vi "USB_TC-08 - Data table 2inputs.vi"() -> ()   [LabVIEW 2018]
uses:
  Instance           1 17Saved   USB_TC-08 .vi
  Program Files (x86)/Pico Technology/SDK/lib/usbtc08.dll
panel:
  in  "Units 3":enum16{"--"}(ring)
  in  "Units 2":enum16{"C°", "F°", "K°", "R°"}(ring)
  out "Temperature 2":dynamicdata(graph)
  in  "Type # 2.8":i16(ring)=107 items=["B"=98, "E"=101, "J"=106, "K"=107, "N"=110, "R"=114, "S"=115, "T"=116, "Voltage"=120]
  in  "Type # 2.7":i16(ring)=107 items=["B"=98, "E"=101, "J"=106, "K"=107, "N"=110, "R"=114, "S"=115, "T"=116, "Voltage"=120]
  in  "Type # 2.6":i16(ring)=107 items=["B"=98, "E"=101, "J"=106, "K"=107, "N"=110, "R"=114, "S"=115, "T"=116, "Voltage"=120]
  in  "Type # 2.5":i16(ring)=107 items=["B"=98, "E"=101, "J"=106, "K"=107, "N"=110, "R"=114, "S"=115, "T"=116, "Voltage"=120]
  in  "Type # 2.4":i16(ring)=107 items=["B"=98, "E"=101, "J"=106, "K"=107, "N"=110, "R"=114, "S"=115, "T"=116, "Voltage"=120]
  in  "Type # 2.3":i16(ring)=107 items=["B"=98, "E"=101, "J"=106, "K"=107, "N"=110, "R"=114, "S"=115, "T"=116, "Voltage"=120]
  in  "Type # 2.2":i16(ring)=107 items=["B"=98, "E"=101, "J"=106, "K"=107, "N"=110, "R"=114, "S"=115, "T"=116, "Voltage"=120]
  in  "Type # 2.1":i16(ring)=107 items=["B"=98, "E"=101, "J"=106, "K"=107, "N"=110, "R"=114, "S"=115, "T"=116, "Voltage"=120]
  in  "Ch # 2.8":bool
  in  "Ch # 2.7":bool
  in  "Ch # 2.6":bool
  in  "Ch # 2.5":bool
  in  "Ch # 2.4":bool
  in  "Ch # 2.3 2":bool
  in  "Ch# 2.2 2":bool=TRUE
  in  "Ch# 2.1":bool=TRUE
  in  "Mains Frequency 2":i16(ring) items=["50 Hz", "60 Hz"]
  out "Handle 2":i16
  in  "?":bool
  in  "Save File Path":path
  in  "Comment":string="WRITE THE COMMENT BEFORE RUNNING VI"
  in  "Save to File":bool
  out "Output Data":string[][](table)
  in  "Mains Frequency":i16(ring) items=["50 Hz", "60 Hz"]
  out "Temperature":dynamicdata(graph)
  in  "?":bool
  in  "Ch # 1.8":bool
  in  "Type # 1.8":i16(ring)=107 items=["B"=98, "E"=101, "J"=106, "K"=107, "N"=110, "R"=114, "S"=115, "T"=116, "Voltage"=120]
  in  "Ch # 1.7":bool
  in  "Type # 1.7":i16(ring)=107 items=["B"=98, "E"=101, "J"=106, "K"=107, "N"=110, "R"=114, "S"=115, "T"=116, "Voltage"=120]
  in  "Ch # 1.6":bool
  in  "Type # 1.6":i16(ring)=107 items=["B"=98, "E"=101, "J"=106, "K"=107, "N"=110, "R"=114, "S"=115, "T"=116, "Voltage"=120]
  in  "Ch # 1.5":bool
  in  "Type # 1.5":i16(ring)=107 items=["B"=98, "E"=101, "J"=106, "K"=107, "N"=110, "R"=114, "S"=115, "T"=116, "Voltage"=120]
  in  "Ch # 1.4":bool
  in  "Type # 1.4":i16(ring)=107 items=["B"=98, "E"=101, "J"=106, "K"=107, "N"=110, "R"=114, "S"=115, "T"=116, "Voltage"=120]
  in  "Ch # 1.3":bool
  in  "Type # 1.3":i16(ring)=107 items=["B"=98, "E"=101, "J"=106, "K"=107, "N"=110, "R"=114, "S"=115, "T"=116, "Voltage"=120]
  in  "Ch# 1.2":bool=TRUE
  in  "Type # 1.2":i16(ring)=107 items=["B"=98, "E"=101, "J"=106, "K"=107, "N"=110, "R"=114, "S"=115, "T"=116, "Voltage"=120]
  in  "Ch# 1.1":bool=TRUE
  in  "Type # 1.1":i16(ring)=107 items=["B"=98, "E"=101, "J"=106, "K"=107, "N"=110, "R"=114, "S"=115, "T"=116, "Voltage"=120]
  in  "Units":enum16{"C°", "F°", "K°", "R°"}(ring)
  in  "stop":bool
  out "Handle":i16
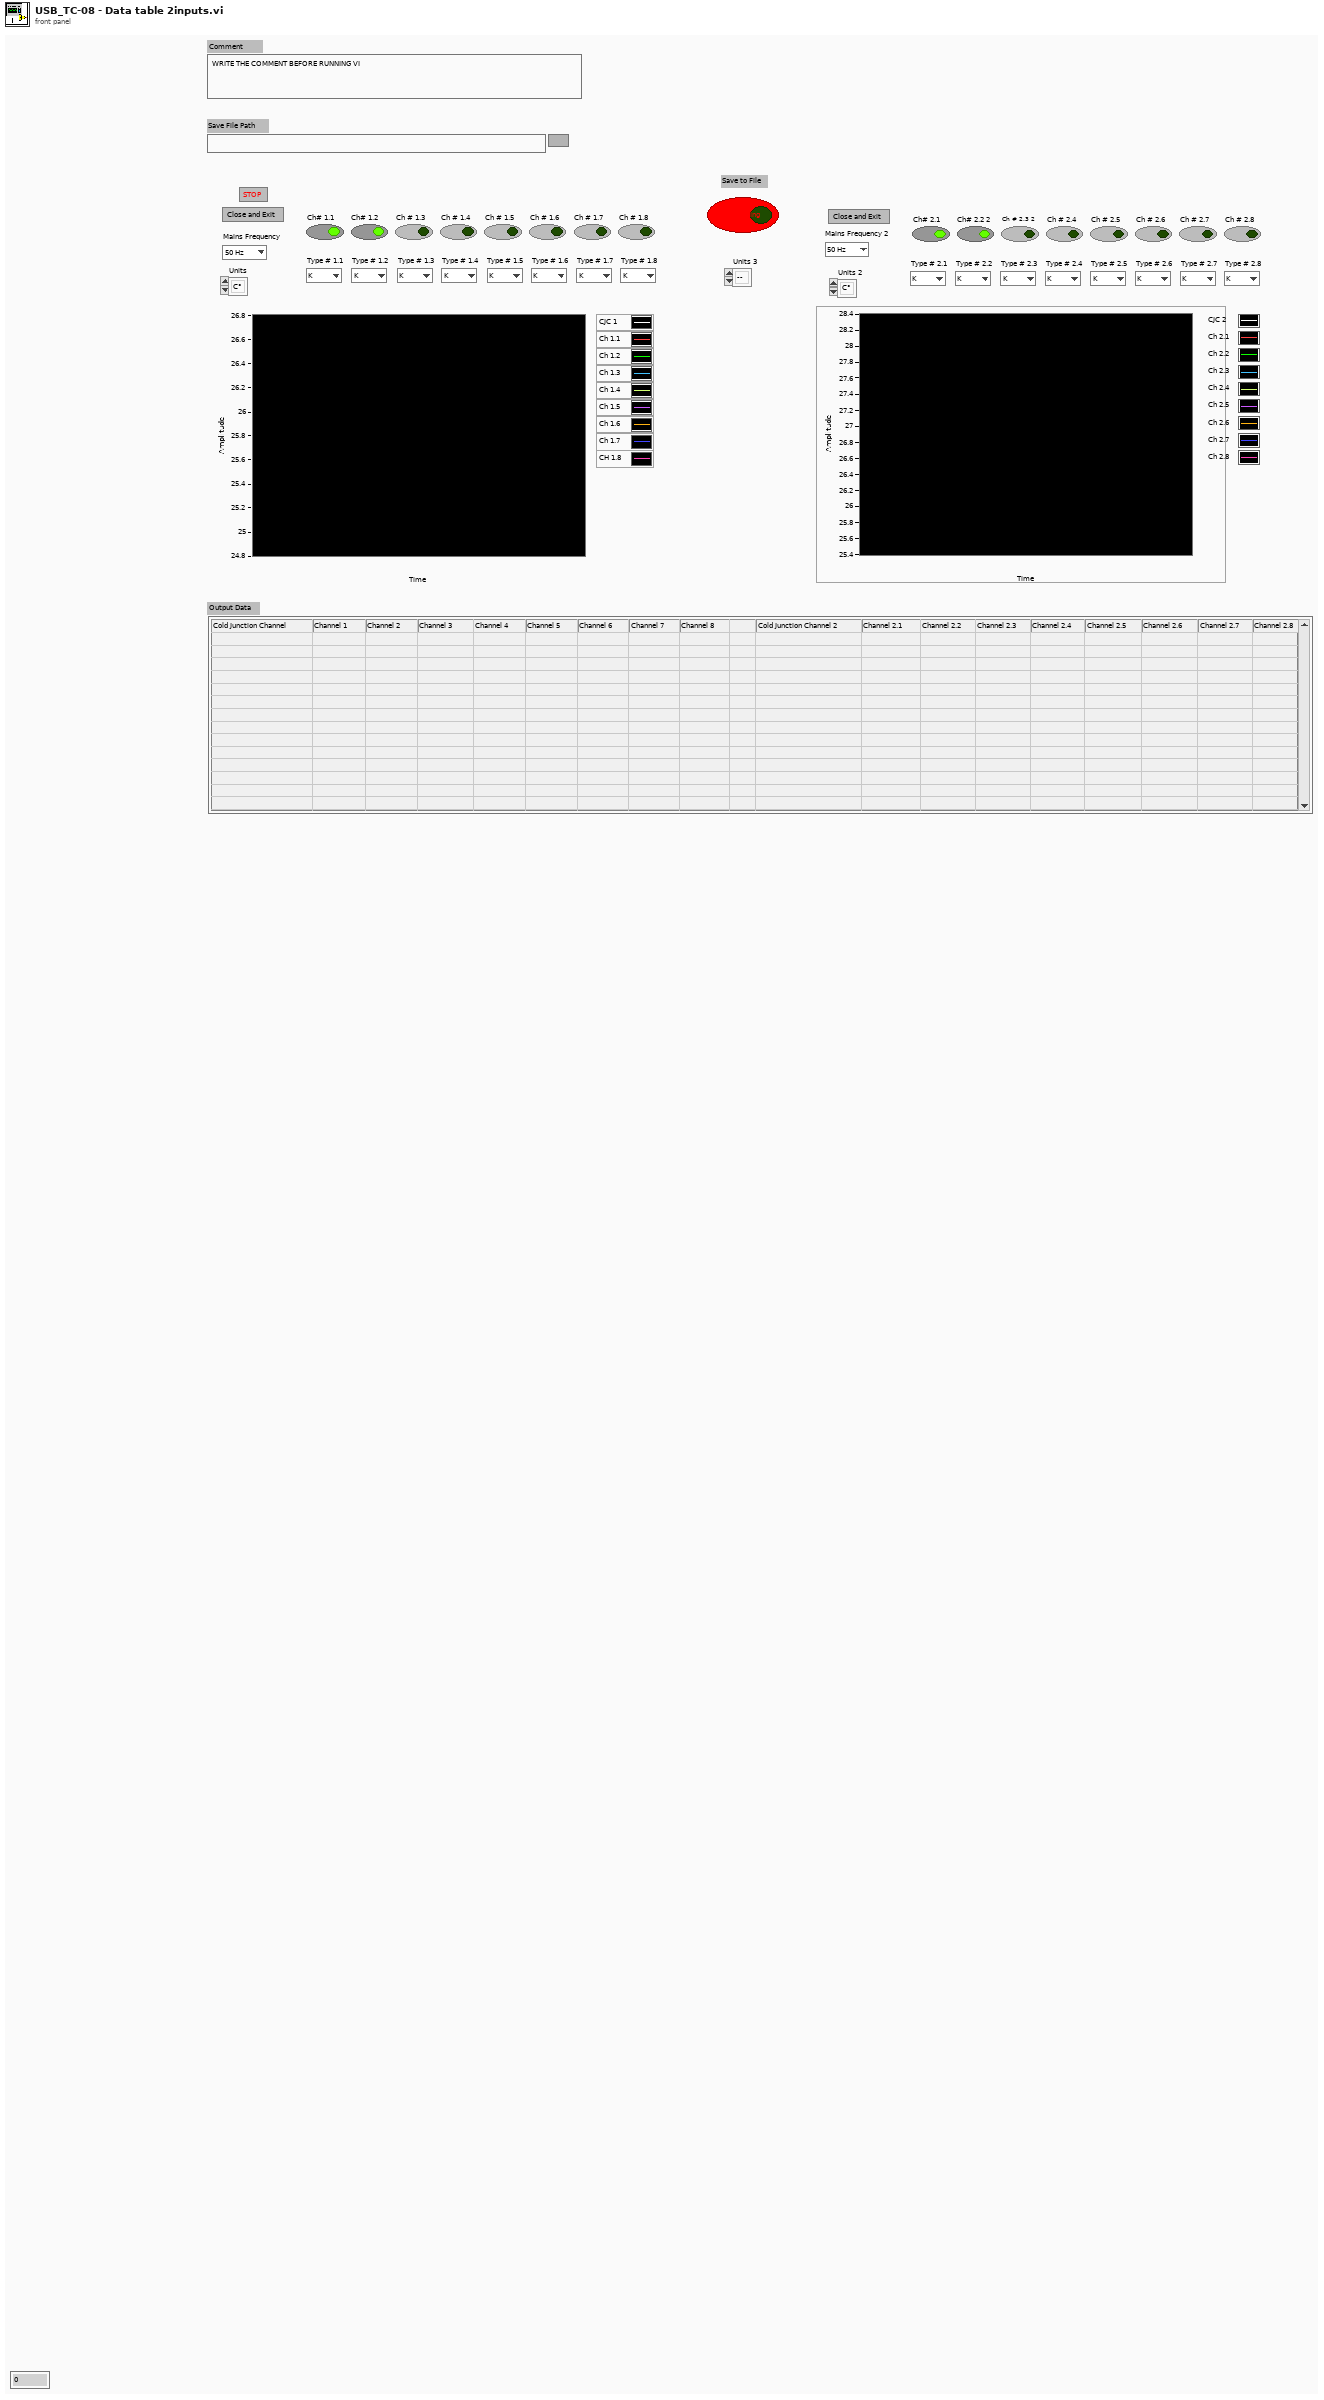
[diagram p1: front panel]
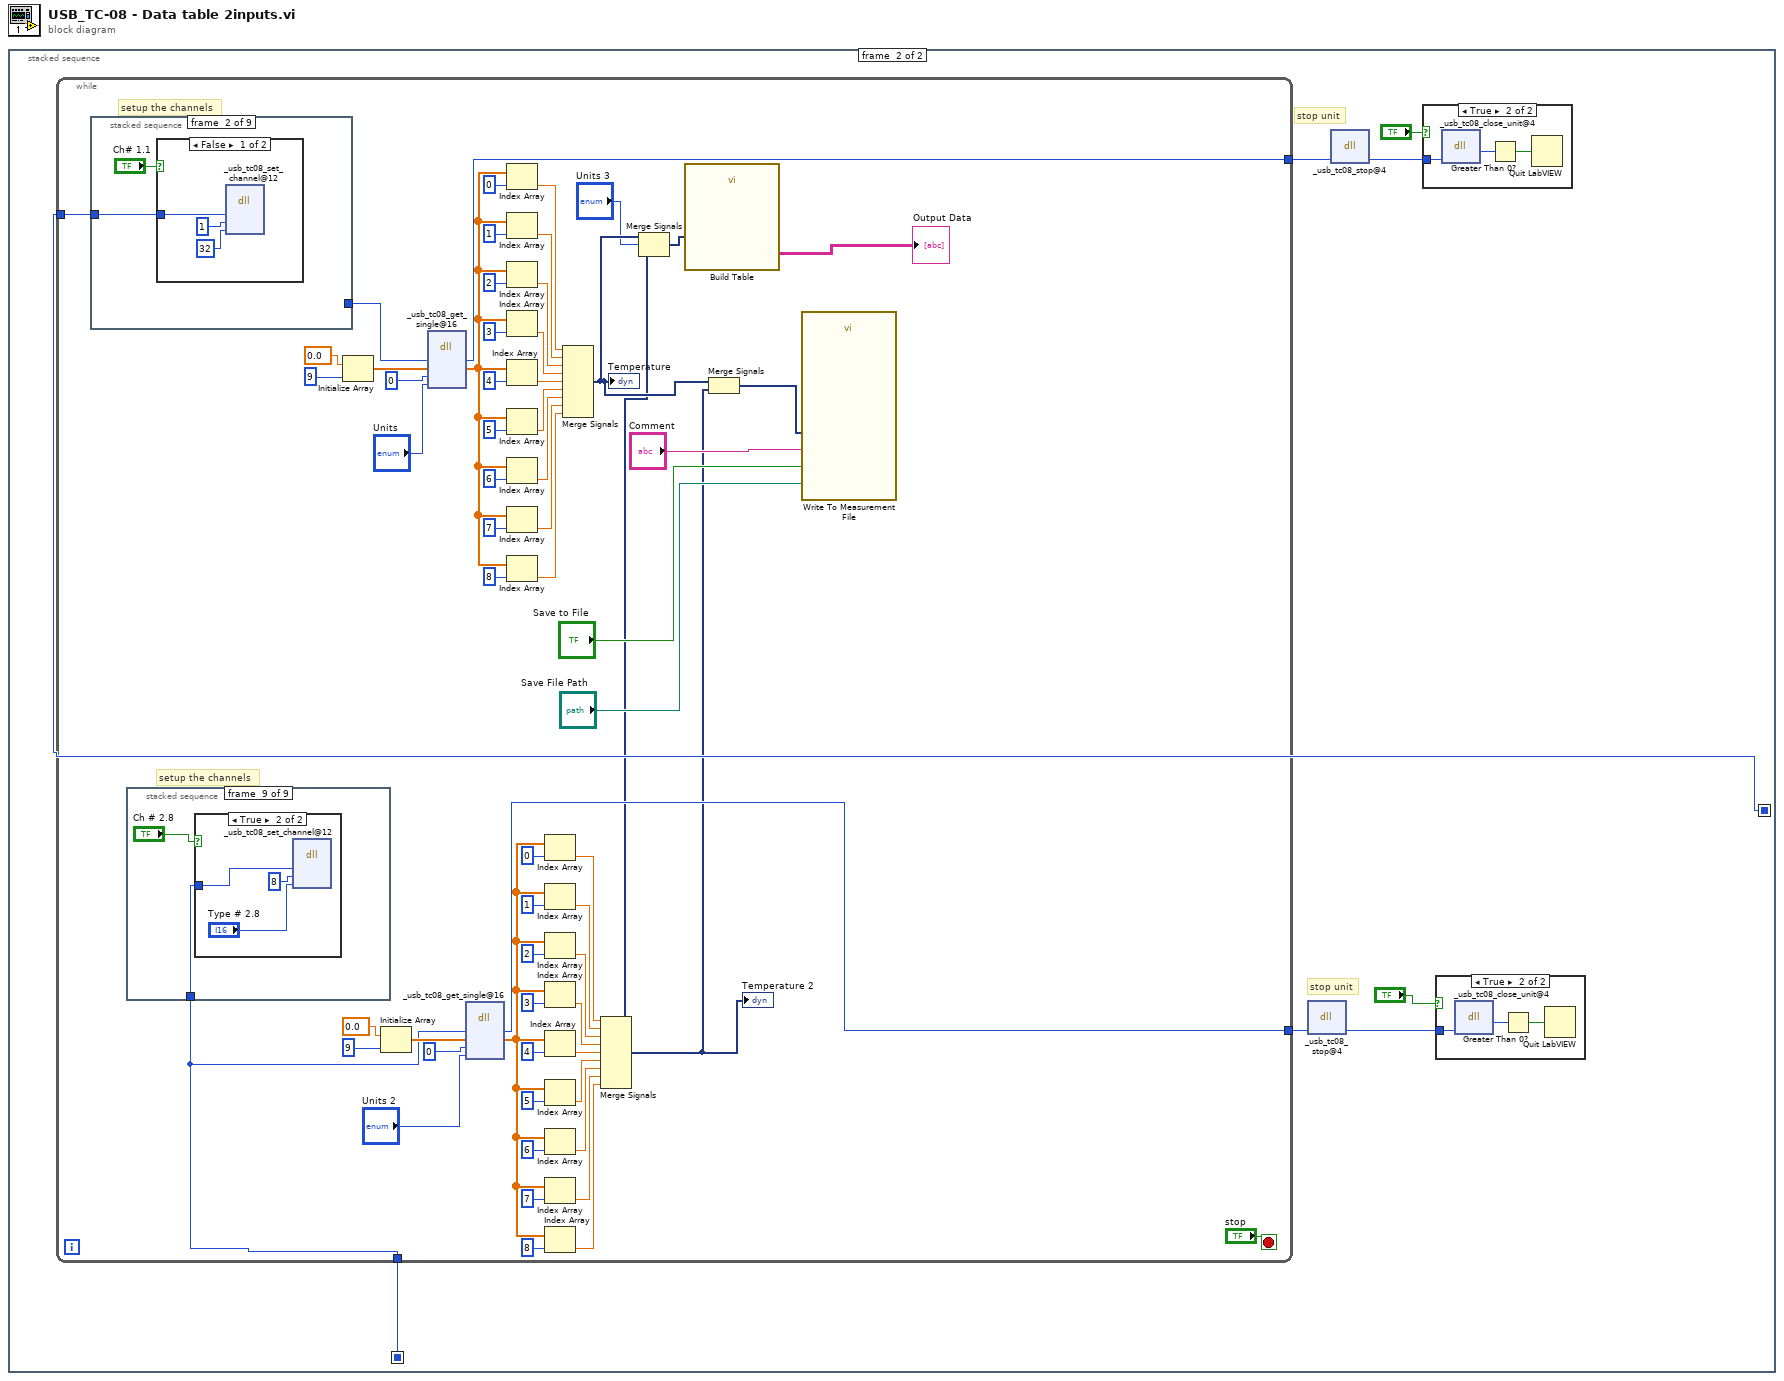
[diagram p0: block diagram]
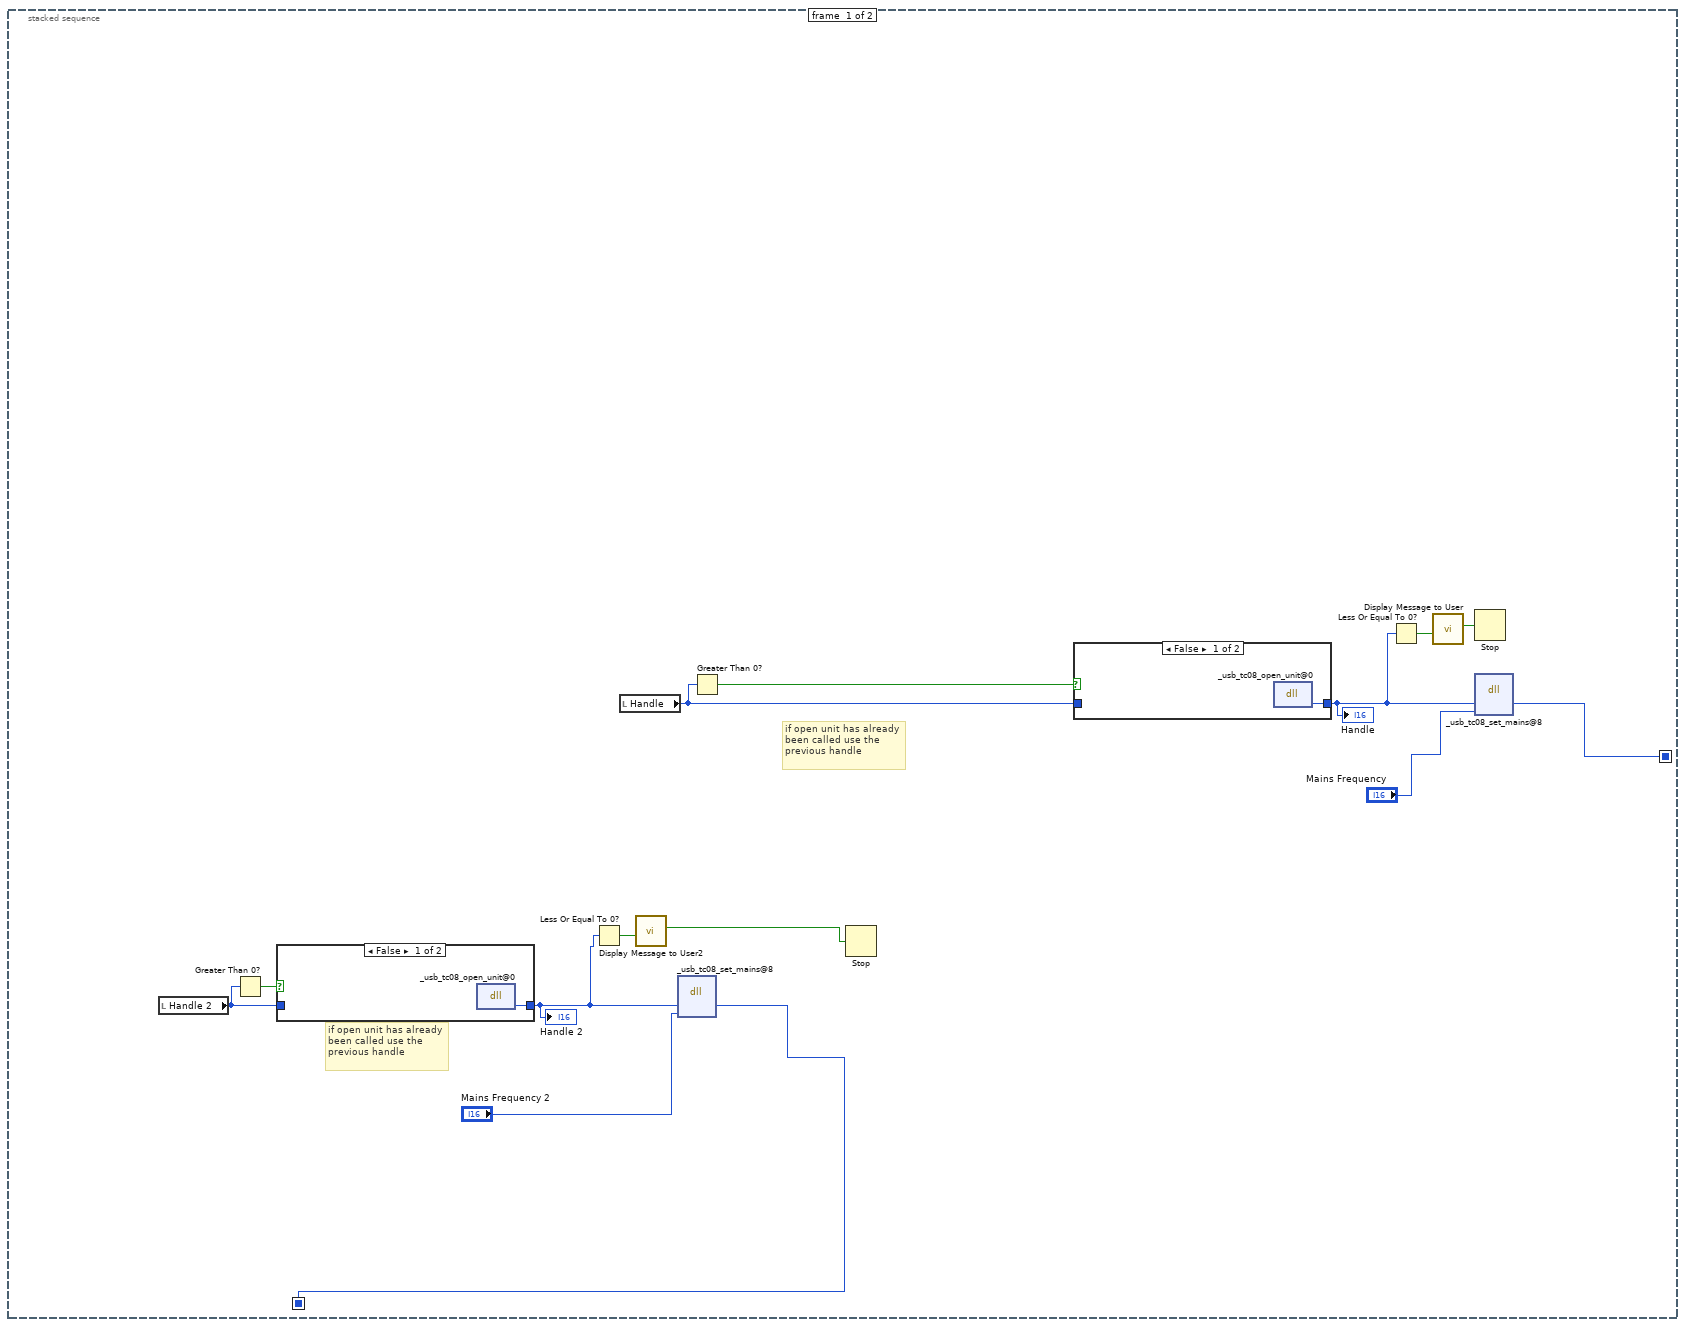
[diagram p2: hidden frame]
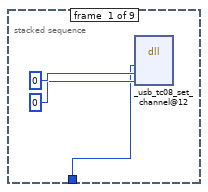
[diagram p6: hidden frame]
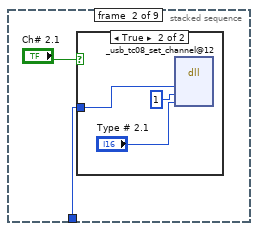
[diagram p7: hidden frame]
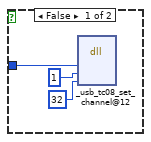
[diagram p8: hidden frame]
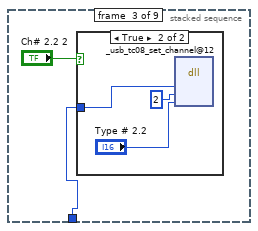
[diagram p9: hidden frame]
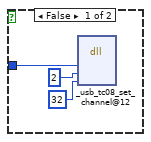
[diagram p10: hidden frame]
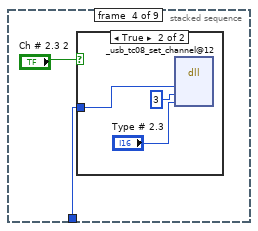
[diagram p11: hidden frame]
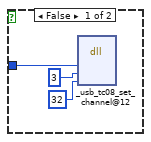
[diagram p12: hidden frame]
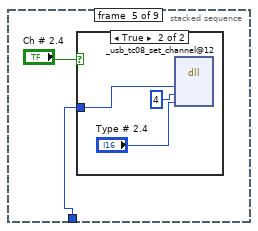
[diagram p13: hidden frame]
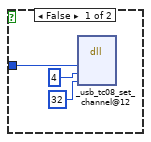
[diagram p14: hidden frame]
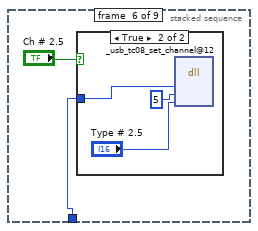
[diagram p15: hidden frame]
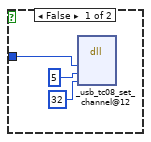
[diagram p16: hidden frame]
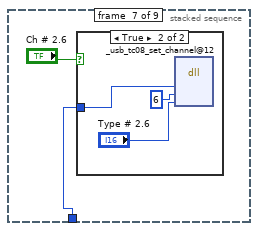
[diagram p17: hidden frame]
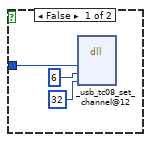
[diagram p18: hidden frame]
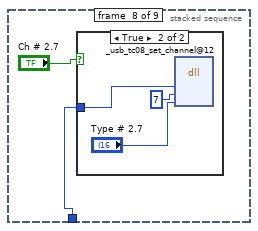
[diagram p19: hidden frame]
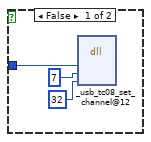
[diagram p20: hidden frame]
diagram:
  n1 = stacked-sequence {
    seq-local: [w12 _] -> [_ w23]
    seq-local: [w1 _] -> [_ w19]
    frame #0 {
      # "if open unit has already been called use the previous handle"
      # "if open unit has already been called use the previous handle"
      n2 = local read "Handle 2"() -> (w6:i16)
      n3 = Greater Than 0?(x=w6) -> (x > 0?=w5:bool)
      n4 = case shown="False" w5 {
        tunnel: [w15 w16] -> w2
        tunnel: w6 -> [_ w16]
        frame False {
          n5 = dll-call lib="//Program Files (x86)/Pico Technology/SDK/lib/usbtc08.dll" fn="_usb_tc08_open_unit@0" label="OpenUnit"() -> ("Handle"=w15:i16)  [unwired: 3 in, 2 out]
        }
        frame True {
        }
      }
      "Handle 2" <- w2
      n6 = Less Or Equal To 0?(x=w2) -> (x <= 0?=w4:bool)
      n7 = local read "Handle"() -> (w13:i16)
      n8 = call "Display Message to User2"("Enable"=w4) -> ("OK"=w3:bool)  [unwired: 9 in, 1 out]
      n9 = dll-call lib="//Program Files (x86)/Pico Technology/SDK/lib/usbtc08.dll" fn="_usb_tc08_set_mains@8" label="Set Mains"("Handle"=w2, "sixtyHertz"="Mains Frequency 2") -> ("Handle"=w1:i16)  [unwired: 5 in, 2 out]
      n10 = Greater Than 0?(x=w13) -> (x > 0?=w14:bool)
      n11 = Stop(stop? (T)=w3) -> ()
      n12 = case shown="False" w14 {
        tunnel: [w17 w18] -> w11
        tunnel: w13 -> [_ w18]
        frame False {
          n13 = dll-call lib="//Program Files (x86)/Pico Technology/SDK/lib/usbtc08.dll" fn="_usb_tc08_open_unit@0" label="OpenUnit"() -> ("Handle"=w17:i16)  [unwired: 3 in, 2 out]
        }
        frame True {
        }
      }
      "Handle" <- w11
      n14 = Less Or Equal To 0?(x=w11) -> (x <= 0?=w10:bool)
      n15 = call "Display Message to User"("Enable"=w10) -> ("OK"=w9:bool)  [unwired: 9 in, 1 out]
      n16 = Stop(stop? (T)=w9) -> ()
      n17 = dll-call lib="//Program Files (x86)/Pico Technology/SDK/lib/usbtc08.dll" fn="_usb_tc08_set_mains@8" label="Set Mains"("Handle"=w11, "sixtyHertz"="Mains Frequency") -> ("Handle"=w12:i16)  [unwired: 5 in, 2 out]
    }
    frame #1 {
      # "stop unit"
      # "stop unit"
      n18 = while {
        tunnel: w23 -> [w92]
        tunnel: [w66] -> w24
        tunnel: [w36] -> w20
        tunnel: w19 -> [w35]
        stop <- "stop" stop-if-true
        # "setup the channels"
        # "setup the channels"
        n19 = stacked-sequence {
          tunnel: w92 -> [w162 w164 w172 w180 w188 w196 w204 w212 w219]
          tunnel: [_ _ _ _ _ _ _ _ w219] -> w88
          frame #0 {
            n20 = dll-call lib="//Program Files (x86)/Pico Technology/SDK/lib/usbtc08.dll" fn="_usb_tc08_set_channel@12"("handle"=w162, "channel"=i16 0, "tc_type"=i8 0) -> ()  [unwired: 7 in, 2 out]
          }
          frame #1 {
            n21 = case shown="False" "Ch# 1.1" {
              tunnel: w164 -> [w166 w169]
              frame False {
                n22 = dll-call lib="//Program Files (x86)/Pico Technology/SDK/lib/usbtc08.dll" fn="_usb_tc08_set_channel@12"("handle"=w166, "channel"=i16 1, "tc_type"=32) -> ()  [unwired: 7 in, 2 out]
              }
              frame True {
                n23 = dll-call lib="//Program Files (x86)/Pico Technology/SDK/lib/usbtc08.dll" fn="_usb_tc08_set_channel@12"("handle"=w169, "channel"=i16 1, "tc_type"="Type # 1.1") -> ()  [unwired: 7 in, 2 out]
              }
            }
          }
          frame #2 {
            n24 = case shown="False" "Ch# 1.2" {
              tunnel: w172 -> [w173 w177]
              frame False {
                n25 = dll-call lib="//Program Files (x86)/Pico Technology/SDK/lib/usbtc08.dll" fn="_usb_tc08_set_channel@12"("handle"=w173, "channel"=i16 2, "tc_type"=32) -> ()  [unwired: 7 in, 2 out]
              }
              frame True {
                n26 = dll-call lib="//Program Files (x86)/Pico Technology/SDK/lib/usbtc08.dll" fn="_usb_tc08_set_channel@12"("handle"=w177, "channel"=i16 2, "tc_type"="Type # 1.2") -> ()  [unwired: 7 in, 2 out]
              }
            }
          }
          frame #3 {
            n27 = case shown="True" "Ch # 1.3" {
              tunnel: w180 -> [w181 w185]
              frame False {
                n28 = dll-call lib="//Program Files (x86)/Pico Technology/SDK/lib/usbtc08.dll" fn="_usb_tc08_set_channel@12"("handle"=w181, "channel"=i16 3, "tc_type"=32) -> ()  [unwired: 7 in, 2 out]
              }
              frame True {
                n29 = dll-call lib="//Program Files (x86)/Pico Technology/SDK/lib/usbtc08.dll" fn="_usb_tc08_set_channel@12"("handle"=w185, "channel"=i16 3, "tc_type"="Type # 1.3") -> ()  [unwired: 7 in, 2 out]
              }
            }
          }
          frame #4 {
            n30 = case shown="False" "Ch # 1.4" {
              tunnel: w188 -> [w189 w193]
              frame False {
                n31 = dll-call lib="//Program Files (x86)/Pico Technology/SDK/lib/usbtc08.dll" fn="_usb_tc08_set_channel@12"("handle"=w189, "channel"=i16 4, "tc_type"=32) -> ()  [unwired: 7 in, 2 out]
              }
              frame True {
                n32 = dll-call lib="//Program Files (x86)/Pico Technology/SDK/lib/usbtc08.dll" fn="_usb_tc08_set_channel@12"("handle"=w193, "channel"=i16 4, "tc_type"="Type # 1.4") -> ()  [unwired: 7 in, 2 out]
              }
            }
          }
          frame #5 {
            n33 = case shown="False" "Ch # 1.5" {
              tunnel: w196 -> [w197 w201]
              frame False {
                n34 = dll-call lib="//Program Files (x86)/Pico Technology/SDK/lib/usbtc08.dll" fn="_usb_tc08_set_channel@12"("handle"=w197, "channel"=i16 5, "tc_type"=32) -> ()  [unwired: 7 in, 2 out]
              }
              frame True {
                n35 = dll-call lib="//Program Files (x86)/Pico Technology/SDK/lib/usbtc08.dll" fn="_usb_tc08_set_channel@12"("handle"=w201, "channel"=i16 5, "tc_type"="Type # 1.5") -> ()  [unwired: 7 in, 2 out]
              }
            }
          }
          frame #6 {
            n36 = case shown="True" "Ch # 1.6" {
              tunnel: w204 -> [w205 w209]
              frame False {
                n37 = dll-call lib="//Program Files (x86)/Pico Technology/SDK/lib/usbtc08.dll" fn="_usb_tc08_set_channel@12"("handle"=w205, "channel"=i16 6, "tc_type"=32) -> ()  [unwired: 7 in, 2 out]
              }
              frame True {
                n38 = dll-call lib="//Program Files (x86)/Pico Technology/SDK/lib/usbtc08.dll" fn="_usb_tc08_set_channel@12"("handle"=w209, "channel"=i16 6, "tc_type"="Type # 1.6") -> ()  [unwired: 7 in, 2 out]
              }
            }
          }
          frame #7 {
            n39 = case shown="False" "Ch # 1.7" {
              tunnel: w212 -> [w213 w217]
              frame False {
                n40 = dll-call lib="//Program Files (x86)/Pico Technology/SDK/lib/usbtc08.dll" fn="_usb_tc08_set_channel@12"("handle"=w213, "channel"=i16 7, "tc_type"=32) -> ()  [unwired: 7 in, 2 out]
              }
              frame True {
                n41 = dll-call lib="//Program Files (x86)/Pico Technology/SDK/lib/usbtc08.dll" fn="_usb_tc08_set_channel@12"("handle"=w217, "channel"=i16 7, "tc_type"="Type # 1.7") -> ()  [unwired: 7 in, 2 out]
              }
            }
          }
          frame #8 {
            n42 = case shown="True" "Ch # 1.8" {
              tunnel: w219 -> [w221 w225]
              frame False {
                n43 = dll-call lib="//Program Files (x86)/Pico Technology/SDK/lib/usbtc08.dll" fn="_usb_tc08_set_channel@12"("handle"=w221, "channel"=i16 8, "tc_type"=32) -> ()  [unwired: 7 in, 2 out]
              }
              frame True {
                n44 = dll-call lib="//Program Files (x86)/Pico Technology/SDK/lib/usbtc08.dll" fn="_usb_tc08_set_channel@12"("handle"=w225, "channel"=i16 8, "tc_type"="Type # 1.8") -> ()  [unwired: 7 in, 2 out]
              }
            }
          }
        }
        n45 = stacked-sequence {
          tunnel: w35 -> [w93 w97 w105 w113 w121 w129 w137 w145 w153]
          frame #0 {
            n46 = dll-call lib="//Program Files (x86)/Pico Technology/SDK/lib/usbtc08.dll" fn="_usb_tc08_set_channel@12"("handle"=w93, "channel"=i16 0, "tc_type"=i8 0) -> ()  [unwired: 7 in, 2 out]
          }
          frame #1 {
            n47 = case shown="True" "Ch# 2.1" {
              tunnel: w97 -> [w99 w102]
              frame False {
                n48 = dll-call lib="//Program Files (x86)/Pico Technology/SDK/lib/usbtc08.dll" fn="_usb_tc08_set_channel@12"("handle"=w99, "channel"=i16 1, "tc_type"=32) -> ()  [unwired: 7 in, 2 out]
              }
              frame True {
                n49 = dll-call lib="//Program Files (x86)/Pico Technology/SDK/lib/usbtc08.dll" fn="_usb_tc08_set_channel@12"("handle"=w102, "channel"=i16 1, "tc_type"="Type # 2.1") -> ()  [unwired: 7 in, 2 out]
              }
            }
          }
          frame #2 {
            n50 = case shown="True" "Ch# 2.2 2" {
              tunnel: w105 -> [w106 w110]
              frame False {
                n51 = dll-call lib="//Program Files (x86)/Pico Technology/SDK/lib/usbtc08.dll" fn="_usb_tc08_set_channel@12"("handle"=w106, "channel"=i16 2, "tc_type"=32) -> ()  [unwired: 7 in, 2 out]
              }
              frame True {
                n52 = dll-call lib="//Program Files (x86)/Pico Technology/SDK/lib/usbtc08.dll" fn="_usb_tc08_set_channel@12"("handle"=w110, "channel"=i16 2, "tc_type"="Type # 2.2") -> ()  [unwired: 7 in, 2 out]
              }
            }
          }
          frame #3 {
            n53 = case shown="True" "Ch # 2.3 2" {
              tunnel: w113 -> [w114 w118]
              frame False {
                n54 = dll-call lib="//Program Files (x86)/Pico Technology/SDK/lib/usbtc08.dll" fn="_usb_tc08_set_channel@12"("handle"=w114, "channel"=i16 3, "tc_type"=32) -> ()  [unwired: 7 in, 2 out]
              }
              frame True {
                n55 = dll-call lib="//Program Files (x86)/Pico Technology/SDK/lib/usbtc08.dll" fn="_usb_tc08_set_channel@12"("handle"=w118, "channel"=i16 3, "tc_type"="Type # 2.3") -> ()  [unwired: 7 in, 2 out]
              }
            }
          }
          frame #4 {
            n56 = case shown="True" "Ch # 2.4" {
              tunnel: w121 -> [w122 w126]
              frame False {
                n57 = dll-call lib="//Program Files (x86)/Pico Technology/SDK/lib/usbtc08.dll" fn="_usb_tc08_set_channel@12"("handle"=w122, "channel"=i16 4, "tc_type"=32) -> ()  [unwired: 7 in, 2 out]
              }
              frame True {
                n58 = dll-call lib="//Program Files (x86)/Pico Technology/SDK/lib/usbtc08.dll" fn="_usb_tc08_set_channel@12"("handle"=w126, "channel"=i16 4, "tc_type"="Type # 2.4") -> ()  [unwired: 7 in, 2 out]
              }
            }
          }
          frame #5 {
            n59 = case shown="True" "Ch # 2.5" {
              tunnel: w129 -> [w130 w134]
              frame False {
                n60 = dll-call lib="//Program Files (x86)/Pico Technology/SDK/lib/usbtc08.dll" fn="_usb_tc08_set_channel@12"("handle"=w130, "channel"=i16 5, "tc_type"=32) -> ()  [unwired: 7 in, 2 out]
              }
              frame True {
                n61 = dll-call lib="//Program Files (x86)/Pico Technology/SDK/lib/usbtc08.dll" fn="_usb_tc08_set_channel@12"("handle"=w134, "channel"=i16 5, "tc_type"="Type # 2.5") -> ()  [unwired: 7 in, 2 out]
              }
            }
          }
          frame #6 {
            n62 = case shown="True" "Ch # 2.6" {
              tunnel: w137 -> [w138 w142]
              frame False {
                n63 = dll-call lib="//Program Files (x86)/Pico Technology/SDK/lib/usbtc08.dll" fn="_usb_tc08_set_channel@12"("handle"=w138, "channel"=i16 6, "tc_type"=32) -> ()  [unwired: 7 in, 2 out]
              }
              frame True {
                n64 = dll-call lib="//Program Files (x86)/Pico Technology/SDK/lib/usbtc08.dll" fn="_usb_tc08_set_channel@12"("handle"=w142, "channel"=i16 6, "tc_type"="Type # 2.6") -> ()  [unwired: 7 in, 2 out]
              }
            }
          }
          frame #7 {
            n65 = case shown="True" "Ch # 2.7" {
              tunnel: w145 -> [w146 w150]
              frame False {
                n66 = dll-call lib="//Program Files (x86)/Pico Technology/SDK/lib/usbtc08.dll" fn="_usb_tc08_set_channel@12"("handle"=w146, "channel"=i16 7, "tc_type"=32) -> ()  [unwired: 7 in, 2 out]
              }
              frame True {
                n67 = dll-call lib="//Program Files (x86)/Pico Technology/SDK/lib/usbtc08.dll" fn="_usb_tc08_set_channel@12"("handle"=w150, "channel"=i16 7, "tc_type"="Type # 2.7") -> ()  [unwired: 7 in, 2 out]
              }
            }
          }
          frame #8 {
            n68 = case shown="True" "Ch # 2.8" {
              tunnel: w153 -> [w154 w158]
              frame False {
                n69 = dll-call lib="//Program Files (x86)/Pico Technology/SDK/lib/usbtc08.dll" fn="_usb_tc08_set_channel@12"("handle"=w154, "channel"=i16 8, "tc_type"=32) -> ()  [unwired: 7 in, 2 out]
              }
              frame True {
                n70 = dll-call lib="//Program Files (x86)/Pico Technology/SDK/lib/usbtc08.dll" fn="_usb_tc08_set_channel@12"("handle"=w158, "channel"=i16 8, "tc_type"="Type # 2.8") -> ()  [unwired: 7 in, 2 out]
              }
            }
          }
        }
        n71 = Initialize Array(sgl 0.0, i16 9) -> (w91:sgl[])
        n72 = Initialize Array(sgl 0.0, i16 9) -> (w37:sgl[])
        n73 = dll-call lib="//Program Files (x86)/Pico Technology/SDK/lib/usbtc08.dll" fn="_usb_tc08_get_single@16"("handle"=w88, "temp_buffer"=w91, "overflow"=i16 0, "units"="Units") -> ("handle"=w66:i16, "temp_buffer"=w76:sgl[])  [unwired: 6 in, 2 out]
        n74 = dll-call lib="//Program Files (x86)/Pico Technology/SDK/lib/usbtc08.dll" fn="_usb_tc08_get_single@16"("handle"=w35, "temp_buffer"=w37, "overflow"=i16 0, "units"="Units 2") -> ("handle"=w36:i16, "temp_buffer"=w50:sgl[])  [unwired: 6 in, 2 out]
        n75 = Index Array(array=w76, index=i16 0) -> (element=w75:sgl)
        n76 = Index Array(array=w76, index=i16 1) -> (element=w65:sgl)
        n77 = Index Array(array=w76, index=i16 2) -> (element=w74:sgl)
        n78 = Index Array(array=w76, index=i16 3) -> (element=w73:sgl)
        n79 = Index Array(array=w76, index=4) -> (element=w72:sgl)
        n80 = Index Array(array=w76, index=i16 5) -> (element=w71:sgl)
        n81 = Index Array(array=w76, index=6) -> (element=w70:sgl)
        n82 = Index Array(array=w76, index=i16 7) -> (element=w68:sgl)
        n83 = Index Array(array=w76, index=i16 8) -> (element=w69:sgl)
        n84 = Index Array(array=w50, index=i16 0) -> (element=w51:sgl)
        n85 = Index Array(array=w50, index=i16 1) -> (element=w59:sgl)
        n86 = Index Array(array=w50, index=i16 2) -> (element=w52:sgl)
        n87 = Index Array(array=w50, index=i16 3) -> (element=w53:sgl)
        n88 = Index Array(array=w50, index=4) -> (element=w54:sgl)
        n89 = Index Array(array=w50, index=i16 5) -> (element=w55:sgl)
        n90 = Index Array(array=w50, index=6) -> (element=w56:sgl)
        n91 = Index Array(array=w50, index=i16 7) -> (element=w58:sgl)
        n92 = Index Array(array=w50, index=i16 8) -> (element=w57:sgl)
        n93 = Merge Signals(w75, w65, w74, w73, w72, w71, w70, w68, w69) -> (w60:dynamicdata)
        "Temperature" <- w60
        n94 = Merge Signals(w51, w59, w52, w53, w54, w55, w56, w58, w57) -> (w31:dynamicdata)
        "Temperature 2" <- w31
        n95 = Merge Signals(w60, "Units 3", w31) -> (w33:dynamicdata)
        n96 = call "Build Table"("Signals"=w33) -> ("Table"=→"Output Data":string[][])  [unwired: 9 in, 1 out]
        n97 = Merge Signals(w60, w31) -> (w34:dynamicdata)
        n98 = call "Write To Measurement File"("Signals"=w34, "Enable"="Save to File", "Filename"="Save File Path", "Comment"="Comment") -> ()  [unwired: 13 in, 3 out]
      }
      n99 = dll-call lib="//Program Files (x86)/Pico Technology/SDK/lib/usbtc08.dll" fn="_usb_tc08_stop@4" ("Close unit")("handle"=w20) -> ("handle"=w22:i16)  [unwired: 4 in, 2 out]
      n100 = dll-call lib="//Program Files (x86)/Pico Technology/SDK/lib/usbtc08.dll" fn="_usb_tc08_stop@4" ("Close unit")("handle"=w24) -> ("handle"=w26:i16)  [unwired: 4 in, 2 out]
      n101 = case shown="True" "?" {
        tunnel: w26 -> [_ w229]
        frame False {
        }
        frame True {
          n102 = dll-call lib="//Program Files (x86)/Pico Technology/SDK/lib/usbtc08.dll" fn="_usb_tc08_close_unit@4" ("Close unit")("handle"=w229) -> (w228:i16)  [unwired: 4 in, 2 out]
          n103 = Greater Than 0?(x=w228) -> (x > 0?=w227:bool)
          n104 = Quit LabVIEW(quit? (T)=w227) -> ()
        }
      }
      n105 = case shown="True" "?" {
        tunnel: w22 -> [_ w29]
        frame False {
        }
        frame True {
          n106 = dll-call lib="//Program Files (x86)/Pico Technology/SDK/lib/usbtc08.dll" fn="_usb_tc08_close_unit@4" ("Close unit")("handle"=w29) -> (w28:i16)  [unwired: 4 in, 2 out]
          n107 = Greater Than 0?(x=w28) -> (x > 0?=w27:bool)
          n108 = Quit LabVIEW(quit? (T)=w27) -> ()
        }
      }
    }
  }
